vi "WSVCAP SHL Host TL RFFE Write Cycle - Multiple DUTs - Common Data.vi"(0 "Data Out (Cycle Commands)":string[](array[string]), 5 "Post Command Delay":dbl[](array[numeric]) format="%#.0p s", 11 "error in":errorcluster, 12 "FPGA":T1, 13 "DUT Mask (All)":bool[](array[boolean])=[TRUE, TRUE, TRUE, TRUE, TRUE, TRUE, TRUE, TRUE, TRUE, TRUE, TRUE, TRUE, TRUE, TRUE, TRUE, TRUE, TRUE, TRUE, TRUE, TRUE, TRUE, TRUE, TRUE, TRUE, TRUE, TRUE, TRUE, TRUE, TRUE, TRUE, TRUE, TRUE, TRUE, TRUE, TRUE, TRUE, TRUE, TRUE, TRUE, TRUE, TRUE, TRUE, TRUE, TRUE, TRUE, TRUE, TRUE, TRUE, TRUE, TRUE, TRUE, TRUE, TRUE, TRUE, TRUE, TRUE, TRUE, TRUE, TRUE, TRUE, TRUE, TRUE, TRUE, TRUE], 14 "Log (T)":bool=TRUE) -> (15 "error out":errorcluster)   [LabVIEW 2017]
uses:
  Type Defs/WSVCAP SHL FPGA Enum.ctl
panel:
  out "Socket Mask":u64=1 format="%02x"
  out "RFFE Data Out [U8]":u8[][](array[numeric]) format="%02x"
  # "DUT 01"
  # "DUT 02"
  # "DUT 03"
  # "DUT 04"
  # "DUT 05"
  # "DUT 06"
  # "DUT 07"
  # "DUT 08"
  # "DUT 09"
  # "DUT 10"
  # "DUT 11"
  # "DUT 12"
  # "DUT 13"
  # "DUT 14"
  # "DUT 15"
  # "DUT 16"
  # "DUT 17"
  # "DUT 18"
  # "DUT 19"
  # "DUT 20"
  # "DUT 21"
  # "DUT 22"
  # "DUT 23"
  # "DUT 24"
  # "DUT 25"
  # "DUT 26"
  # "DUT 27"
  # "DUT 28"
  # "DUT 29"
  # "DUT 30"
  # "DUT 31"
  # "DUT 32"
  # "DUT 33"
  # "DUT 34"
  # "DUT 35"
  # "DUT 36"
  # "DUT 37"
  # "DUT 38"
  # "DUT 39"
  # "DUT 40"
  # "DUT 41"
  # "DUT 42"
  # "DUT 43"
  # "DUT 44"
  # "DUT 45"
  # "DUT 46"
  # "DUT 47"
  # "DUT 48"
  # "DUT 49"
  # "DUT 50"
  # "DUT 51"
  # "DUT 52"
  # "DUT 53"
  # "DUT 54"
  # "DUT 55"
  # "DUT 56"
  # "DUT 57"
  # "DUT 58"
  # "DUT 59"
  # "DUT 60"
  # "DUT 61"
  # "DUT 62"
  # "DUT 63"
  # "DUT 64"
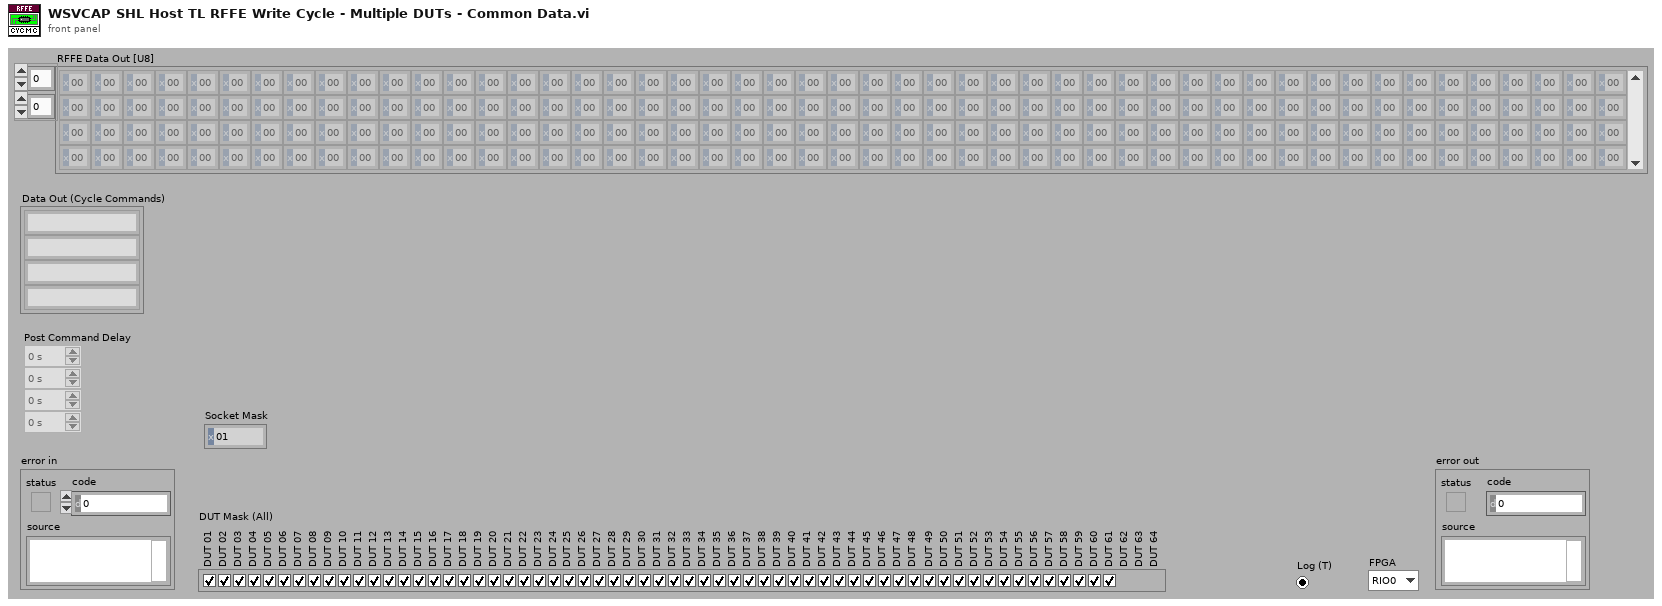
[diagram p1: front panel]
types:
  T1 = typedef "WSVCAP SHL FPGA Enum.ctl" = enum16{"RIO0", "RIO1"}
  T2 = typedef "WSVCAP SHL Core System Cluster.ctl" = cluster{"Settings":T3, "FPGA Resource":tag, "Online":bool, "I2C Wait Ticks":u32, "SPI Wait Ticks":u32, "RFFE Wait Ticks":u32, "FPGA VI Reference (FPGA Mode)":T4, "FPGA VI Reference (Sim Mode)":refnum<vi>}
  T3 = typedef "WSVCAP SHL I2C Settings Cluster.ctl" = cluster{"I2C Slave Address":u8, "I2C Clock Rate (Hz)":dbl, "SPI Clock Rate (Hz)":dbl, "RFFE Slave Address":u8, "RFFE Clock Rate (Hz)":dbl, "Simulate FPGA":bool, "C1 Cap DAC Default":u8, "C2 Cap DAC Default":u8, "C3 Cap DAC Default":u8, "C4 Cap DAC Default":u8}
  T4 = typedef "WSVCAP SHL FPGA Ref.ctl" = refnum<k20>
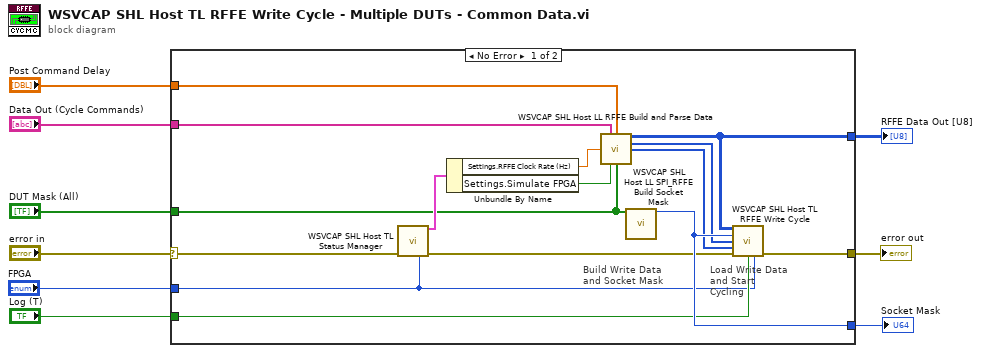
[diagram p0: block diagram]
diagram:
  n1 = case shown="No Error" "error in" {
    selector: "error in" -> [w10 _]
    tunnel: [w24 _] -> w9
    tunnel: [w23 _] -> w7
    tunnel: [w22 _] -> w6
    tunnel: "DUT Mask (All)" -> [w13 _]
    tunnel: "Post Command Delay" -> [w21 _]
    tunnel: "Data Out (Cycle Commands)" -> [w20 _]
    tunnel: "Log (T)" -> [w12 _]
    tunnel: "FPGA" -> [w11 _]
    frame No Error {
      # "Load Write Data and Start Cycling"
      # "Build Write Data and Socket Mask"
      n2 = call "WSVCAP SHL Host TL Status Manager.vi"("error in"=w10, "FPGA"=w11) -> ("System Out"=w19:T2, "error out"=w18:errorcluster)  [unwired: 12 in]
      n3 = Unbundle By Name(w19) -> ("Settings.RFFE Clock Rate (Hz)"=w14:dbl, "Settings.Simulate FPGA"=w17:bool)
      n4 = call "WSVCAP SHL Host LL RFFE Build and Parse Data.vi"("Data Out (Cycle Commands)"=w20, "Post Command Delay"=w21, "Clock Rate (Hz) (Cycle Only)"=w14, "Simulate FPGA (Cycle Only)"=w17, "DUT Mask (All)"=w13) -> ("RFFE Data Out [U8]"=w23:u8[][], "CMD Lengths (Bits)"=w16:u8[], "CMD Delays (Ticks)"=w15:u32[])  [unwired: 7 in, 1 out]
      n5 = call "WSVCAP SHL Host LL SPI_RFFE Build Socket Mask.vi"("DUT Mask"=w13) -> ("Socket Mask [U64]"=w22:u64)  [unwired: 14 in]
      n6 = call "WSVCAP SHL Host TL RFFE Write Cycle.vi"("RFFE Data Out"=w23, "Socket Mask"=w22, "Cycle CMD Lengths (bits)"=w16, "Cycle CMD Delay (ticks)"=w15, "error in"=w18, "Log (T)"=w12, "FPGA"=w11) -> ("error out"=w24:errorcluster)  [unwired: 8 in]
    }
    frame Error {
    }
  }
  "error out" <- w9
  "RFFE Data Out [U8]" <- w7
  "Socket Mask" <- w6
